vi "CoMP-S Global.vi"() -> ()   [LabVIEW 2014]
panel:
  out "Wavelength Offsets":dbl[][](array[numeric])=[[0.16, -0.01, 0.0, 0.02, 0.02, 0.104, 0.082, 0.14, 0.14, 0.14], [0.184, -0.006, 0.008, 0.044, 0.028, 0.074, 0.106, 0.178, 0.12, 0.12], [0.128, 0.0, 0.0, 0.0, 0.0, 0.0, 0.0, 0.0, -0.044, -0.05], [0.12, -0.036, -0.05, 0.04, 0.026, 0.036, 0.092, 0.15, 0.03, 0.03]] format="%_6e"
  out "Wavelength Slopes":dbl[][](array[numeric])=[[1.085854, 1.047898, 1.026208, 1.014553, 1.0, 0.9551623, 0.9465661, 0.9159018, 0.9189034, 0.9160777], [1.037987, 1.022404, 1.003964, 0.9857455, 1.0, 0.9425763, 0.9342777, 0.8998557, 0.8895401, 0.8873311], [0.8703129, 1.035226, 0.9906089, 0.991796, 1.0, 0.9657027, 0.9764769, 0.917473, 0.8896891, 0.8748796], [1.089982, 1.048058, 1.038468, 1.008325, 1.0, 0.9586574, 0.9448586, 0.9220822, 0.9213725, 0.9177798]] format="%_6e"
  out "Wavelength Intercepts":dbl[][](array[numeric])=[[-8053.743, -3677.076, -4575.486, -7242.226, 0.0, 37.1621, -1653.452, 5871.693, 4282.25, 9049.384], [46194.43, 38139.1, 40268.94, 16970.22, -0.007450581, 32826.53, 13769.53, 50808.23, 77250.35, 92830.64], [857889.7, -8037.925, 144119.1, 37468.25, 0.0, -44692.22, -114423.6, 43945.85, 168658.3, 240359.1], [-18156.21, -8043.795, -5531.646, 2033.314, 0.0, -2158.053, 9842.112, 14347.07, 17298.31, 22238.85]] format="%_6e"
  out "Fit Coefficients":dbl[][](array[numeric])=[[535275.8, 1247.046, 0.6008217, 0.9089022, -0.9009574, 1.103208, -1.395392], [2141076.0, 1315.758, 0.6891061, 0.9986409, -0.8035493, 1.096223, -1.175382], [4251795.0, 1281.261, -0.04732143, 0.4250576, -1.665187, 1.147521, -2.929266], [1064466.0, 1258.277, 0.6967535, 0.8840143, -0.7928057, 1.096236, -1.010414]] format="%_6e"
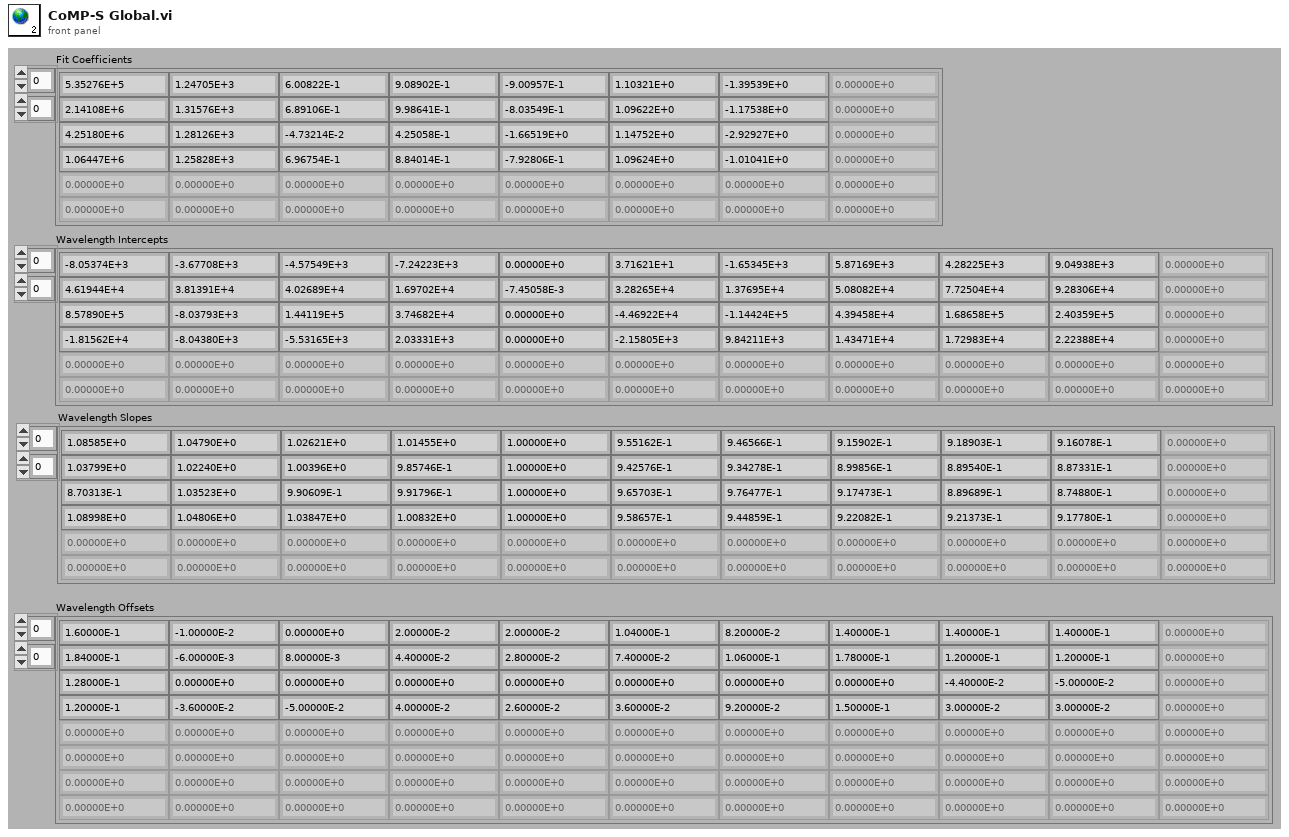
[diagram p1: front panel]
diagram:
